vi "Move Slit Relative Inner.vi"(7 "Mono System # (0)":T2, 8 "error in (no error)":errorcluster, 9 "Steps to Move":i32, 10 "Slit (Front/Axial Entrance)":T1, 11 "VISA resource name":refnum<visa-resource-name>) -> (0 "error out":errorcluster, 3 "VISA resource name out":refnum<visa-resource-name>)   [LabVIEW 2017, in "JY-SPEX-TRIAX.lvlib"]
doc: "Moves the spectrometer's slits a relative number of steps from their current position. Returns control immediately (before the slits are done moving).\n\nA positive number of steps opens the slits wider, while a negative makes them narrower. Note that this command does not correct for backlash; that must be done manually.\n\nOnly one stepper motor can move at a time; thus, this command waits if either other slits or the wavelength drive are being moved.\n\nThe limit to the number of steps that can be moved is the total number of possible steps for the slit."
uses:
  JY-SPEX-TRIAX.lvlib
  controls.llb/Monochromator System Number.ctl
  controls.llb/Slits.ctl
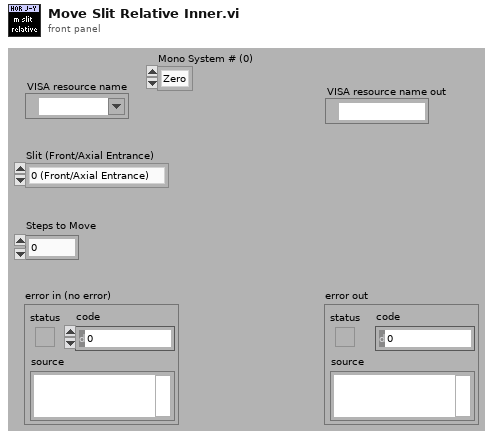
[diagram p1: front panel]
types:
  T1 = typedef "JY-SPEX-TRIAX.lvlib/Slits.ctl" = enum16{"0 (Front/Axial Entrance)", "1 (Side/Lateral Entrance)", "2 (Front/Axial Exit)", "3 (Side/Lateral Exit)"}
  T2 = typedef "JY-SPEX-TRIAX.lvlib/Monochromator System Number.ctl" = enum16{"Zero", "One"}
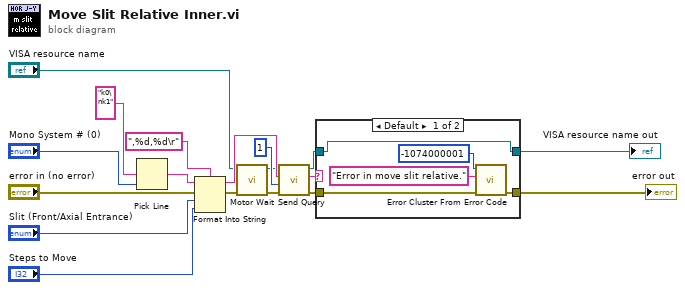
[diagram p0: block diagram]
diagram:
  n1 = Pick Line(multi-line string="k0\nk1", line index="Mono System # (0)") -> (output string=w16:string)  [unwired: 1 out]
  n2 = Format Into String(format string=",%d,%d\r", initial string=w16, error in="error in (no error)", "Slit (Front/Axial Entrance)", "Steps to Move") -> (resulting string=w14:string, error out=w4:errorcluster)
  n3 = call "Motor Wait.vi"("error in"=w4, "VISA resource name in"="VISA resource name") -> ("error out"=w3:errorcluster, "VISA resource name out"=w5:refnum<visa-resource-name>)  [unwired: 8 out]
  n4 = call "Send Query.vi"("error in (no error)"=w3, "byte count"=u32 1, "write buffer"=w14, "VISA resource name"=w5) -> ("error out"=w8:errorcluster, "read buffer"=w10:string, "VISA resource name out"=w9:refnum<visa-resource-name>)  [unwired: 5 out]
  n5 = case shown="Default" w10 {
    tunnel: w9 -> [w19 w25]
    tunnel: [w19 w25] -> w2
    tunnel: w8 -> [w21 w24]
    tunnel: [w20 w24] -> w1
    frame Default {
      n6 = call <vilib>:"Error Cluster From Error Code.vi"("error in (no error)"=w21, "error message (\"\")"="Error in move slit relative." ("error message (\"\")"), "error code (0)"=-1074000001) -> ("error out"=w20:errorcluster)  [unwired: 1 in, 5 out]
    }
    frame "o" {
    }
  }
  "VISA resource name out" <- w2
  "error out" <- w1
